vi "get_sampling_rate.vi"(8 "error in (no error)":errorcluster, 11 "GenericWriteSignals in":refnum<class "GenericSignalWriter.lvclass">) -> (0 "error out":errorcluster, 1 "sampling rate (Hz)":dbl, 2 "sampling rate":dbl[unit], 3 "GenericWriteSignals out":refnum<class "GenericSignalWriter.lvclass">)   [LabVIEW 2010, in "GenericSignalWriter.lvclass"]
uses:
  GenericSignalWriter.lvclass
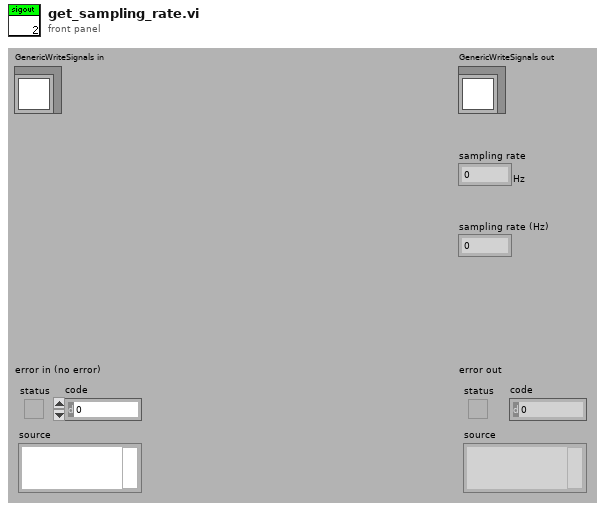
[diagram p1: front panel]
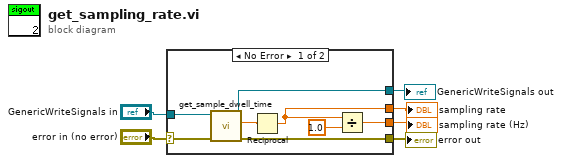
[diagram p0: block diagram]
diagram:
  n1 = case shown="No Error" "error in (no error)" {
    selector: "error in (no error)" -> [w14 w16]
    tunnel: [w13 w16] -> w5
    tunnel: [w11 w15] -> w3
    tunnel: "GenericWriteSignals in" -> [w12 w15]
    tunnel: [w9 _] -> w2
    tunnel: [w7 _] -> w1
    frame No Error {
      n2 = call-dynamic "get_sample_dwell_time.vi"("error in (no error)"=w14, "GenericWriteSignals.lvclass in"=w12) -> ("error out"=w13:errorcluster, "sample dwell time"=w10:dbl[unit], "GenericWriteSignals.lvclass out"=w11:refnum<class "GenericSignalWriter.lvclass">)  [unwired: 7 out]
      n3 = Reciprocal(x=w10) -> (1/x=w9:dbl[unit])
      n4 = Divide(x=w9, y=dbl[unit] 1.0) -> (x/y=w7:dbl)
    }
    frame Error {
    }
  }
  "error out" <- w5
  "GenericWriteSignals out" <- w3
  "sampling rate" <- w2
  "sampling rate (Hz)" <- w1
